vi "Main.vi"() -> ()   [LabVIEW 2018]
doc: "The myRIO Project template acquires acceleration data from the onboard accelerometer and displays the changes of acceleration values in a waveform chart."
uses:
  <vilib>/myRIO/Instrument Drivers/Onboard IO/UART/typedef/VISA Configuration.ctl
  <vilib>/myRIO/Common/Instrument Driver Framework/myRIO v1.0/UART/vis/myRIO v1.0 Close UART.vi
  <vilib>/Instr/_visa.llb/VISA Configure Serial Port (Instr).vi
  <vilib>/myRIO/Common/Instrument Driver Framework/Utilities/vis/FPGA Ref Manager.vi
  <vilib>/myRIO/Common/Instrument Driver Framework/myRIO v1.0/myRIO v1.0 Reset FPGA.vi
  <vilib>/myRIO/Common/Instrument Driver Framework/myRIO v1.0/IRQ/vis/myRIO v1.0 IRQ Info FGV.vi
  <vilib>/myRIO/Common/Instrument Driver Framework/myRIO v1.0/IRQ/vis/myRIO v1.0 Timer IRQ Info FGV.vi
  <vilib>/myRIO/Common/Instrument Driver Framework/myRIO v1.0/IRQ/vis/myRIO v1.0 ISR Agent.vi
  <vilib>/myRIO/Instrument Drivers/Utilities/Utilities.lvlib
  <vilib>/myRIO/Instrument Drivers/Onboard IO/UART/UART.lvlib
panel:
  out "God måling?":bool
  out "Distance [cm]":dbl
  out "Read buffer":string
  out "error out":errorcluster
  in  "Stop":bool
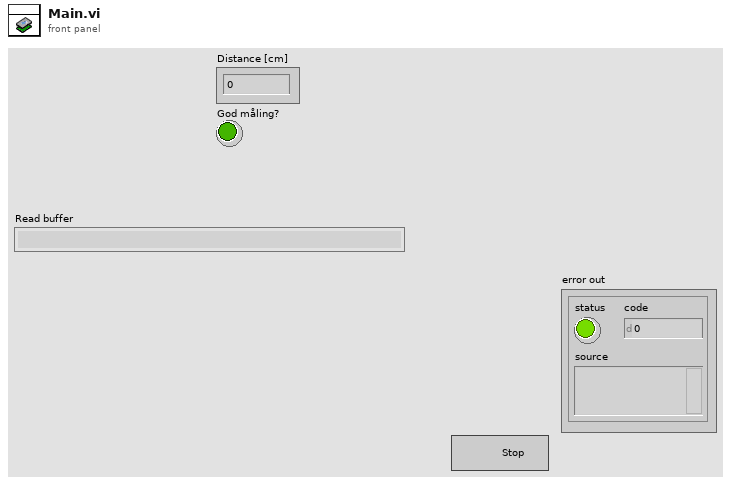
[diagram p1: front panel]
types:
  T1 = typedef "UART.lvlib/VISA Configuration.ctl" = cluster{"baud rate (9600)":u32, "data bits (8)":u16, "parity (0:none)":enum16{"None", "Odd", "Even", "Mark", "Space"}, "stop bits (10: 1 bit)":u16, "flow control (0:none)":u16, "termination char\n(0xA = '\\n' = LF) ":u8, "Enable Termination\nChar (T)":bool, "timeout (10sec)":u32}
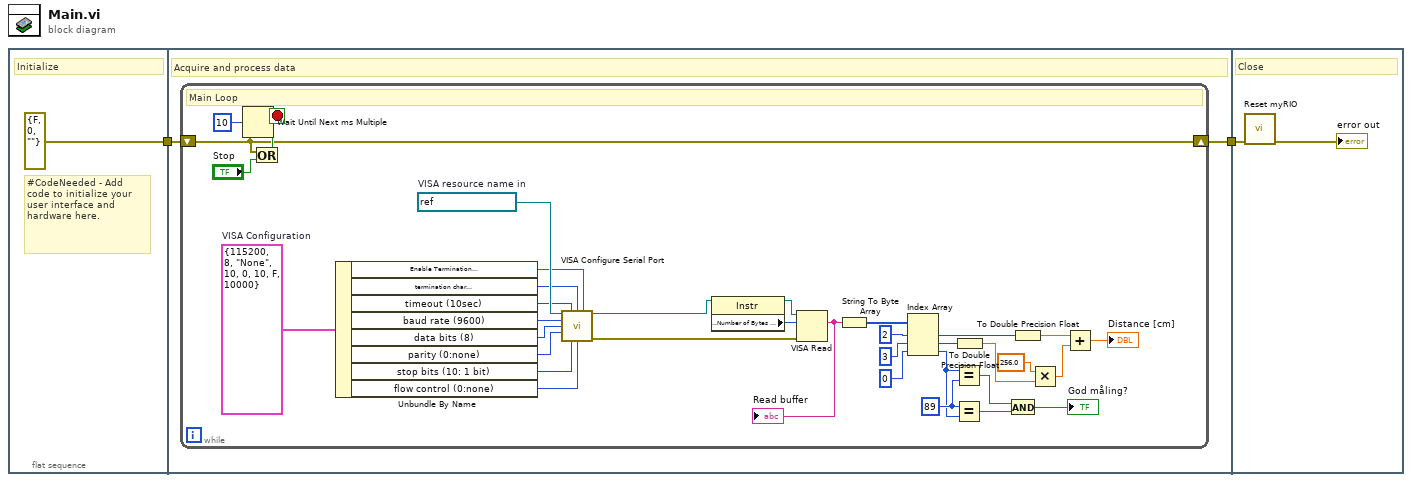
[diagram p0: block diagram]
diagram:
  n1 = flat-sequence {
    tunnel: [errorcluster {"status"=FALSE, "code"=0, "source"=""} ("error in (no error)")] -> w2
    tunnel: w2 -> [w5]
    tunnel: [w4] -> w1
    tunnel: w1 -> [w42]
    frame #0 {
      # "#CodeNeeded - Add code to initialize your user interface and hardware here."
      # "Initialize"
    }
    frame #1 {
      # "Acquire and process data"
      n2 = while {
        shift-right: [w37] -> w4
        shift-left: w5 -> [w37]
        stop <- w39 stop-if-true
        w7 = u8 89 ("y")
        w35 = T1 {"baud rate (9600)"=115200, "data bits (8)"=8, "parity (0:none)"=enum."None", "stop bits (10: 1 bit)"=10, "flow control (0:none)"=0, "termination char\n(0xA = '\\n' = LF) "=10, "Enable Termination\nChar (T)"=FALSE, "timeout (10sec)"=10000}  # VISA Configuration
        w36 = refnum<visa-resource-name> "ASRL1::INSTR"  # VISA resource name in
        # "Main Loop"
        n3 = Wait Until Next ms Multiple(millisecond multiple=u32 10) -> ()  [unwired: 1 out]
        n4 = Or(x=w37, y="Stop") -> (x .or. y?=w39:bool)
        n5 = Unbundle By Name(w35) -> ("Enable Termination\nChar (T)"=w32:bool, "termination char\n(0xA = '\\n' = LF)"=w31:u8, "timeout (10sec)"=w30:u32, "baud rate (9600)"=w25:u32, "data bits (8)"=w26:u16, "parity (0:none)"=w27:enum16{"None", "Odd", "Even", "Mark", "Space"}, "stop bits (10: 1 bit)"=w28:u16, "flow control (0:none)"=w29:u16)
        n6 = call-poly "VISA Configure Serial Port"("VISA resource name"=w36, "timeout (10sec)"=w30, "termination char\n(0xA = '\\n' = LF)"=w31, "Enable Termination\nChar (T)"=w32, "baud rate (9600)"=w25, "data bits (8)"=w26, "parity (0:none)"=w27, "stop bits (10: 1 bit)"=w28, "flow control (0:none)"=w29) -> ("VISA resource name out"=w34:refnum<visa-resource-name>, "error out"=w33:errorcluster)  [unwired: 5 in]
        n7 = property class="Instr"(reference=w34) -> (reference out=w23:refnum<visa-resource-name>, "Serial Settings:Number of Bytes at Serial Port"=w24:u32)  [unwired: 1 in, 1 out]
        n8 = VISA Read(VISA resource name=w23, byte count=w24, error in (no error)=w33) -> (read buffer=w22:string)  [unwired: 3 out]
        "Read buffer" <- w22
        n9 = String To Byte Array(string=w22) -> (unsigned byte array=w21:u8[])
        n10 = Index Array(array=w21, index #1=2 ("index"), index #2=3 ("index"), index #3=0 ("index")) -> (element #1=w16:u8, element #2=w17:u8, element #3=w6:u8)
        n11 = Equal?(x=w6, y=w7) -> (x = y?=w10:bool)
        n12 = Equal?(x=w7, y=w6) -> (x = y?=w9:bool)
        n13 = To Double Precision Float(number=w17) -> (double precision float=w15:dbl)
        n14 = And(x=w10, y=w9) -> (x .and. y?=→"God måling?":bool)
        n15 = To Double Precision Float(number=w16) -> (double precision float=w12:dbl)
        n16 = Multiply(x=256.0, y=w15) -> (x*y=w13:dbl)
        n17 = Add(x=w12, y=w13) -> (x+y=→"Distance [cm]":dbl)
      }
    }
    frame #2 {
      # "Close"
      n18 = call <vilib>:"Reset myRIO.vi"("error in (no error)"=w42) -> ("error out"=→"error out":errorcluster)  [unwired: 10 in]
    }
  }
